vi "Draw Shade.vi"(8 "error in (no error)":errorcluster, 11 "ScrollingList in":refnum<class "ScrollingList.lvclass">) -> (0 "error out":errorcluster, 3 "ScrollingList out":refnum<class "ScrollingList.lvclass">)   [LabVIEW 2020, in "ScrollingList.lvclass"]
uses:
  ScrollingList.lvclass
  C:/Program Files/National Instruments/LabVIEW 2020/vi.lib/QSI/QControls/QControl Classes/Picture/Picture.lvclass
  ScrollingList.lvclass/ScrollingList.ctl
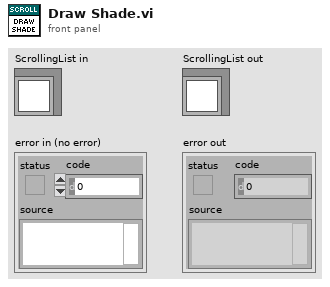
[diagram p1: front panel]
types:
  T1 = cluster{"left":i16, "top":i16, "right":i16, "bottom":i16}
  T2 = cluster{"Width":u16, "Style":enum32{"Solid", "Dash", "Dot", "DashDot", "DashDotDot"}}
  T3 = typedef "ScrollingList.lvclass/State Data.ctl" = cluster{"Timeout":i32, "Time":timestamp, "Y":i32, "Origin:Top":i16, "Rate":dbl, "ListItems":string[], "Item Height":i32, "Max Height":i32}
  T4 = typedef "LVBoundsTypeDef.ctl" = cluster{"Width":u32, "Height":u32}
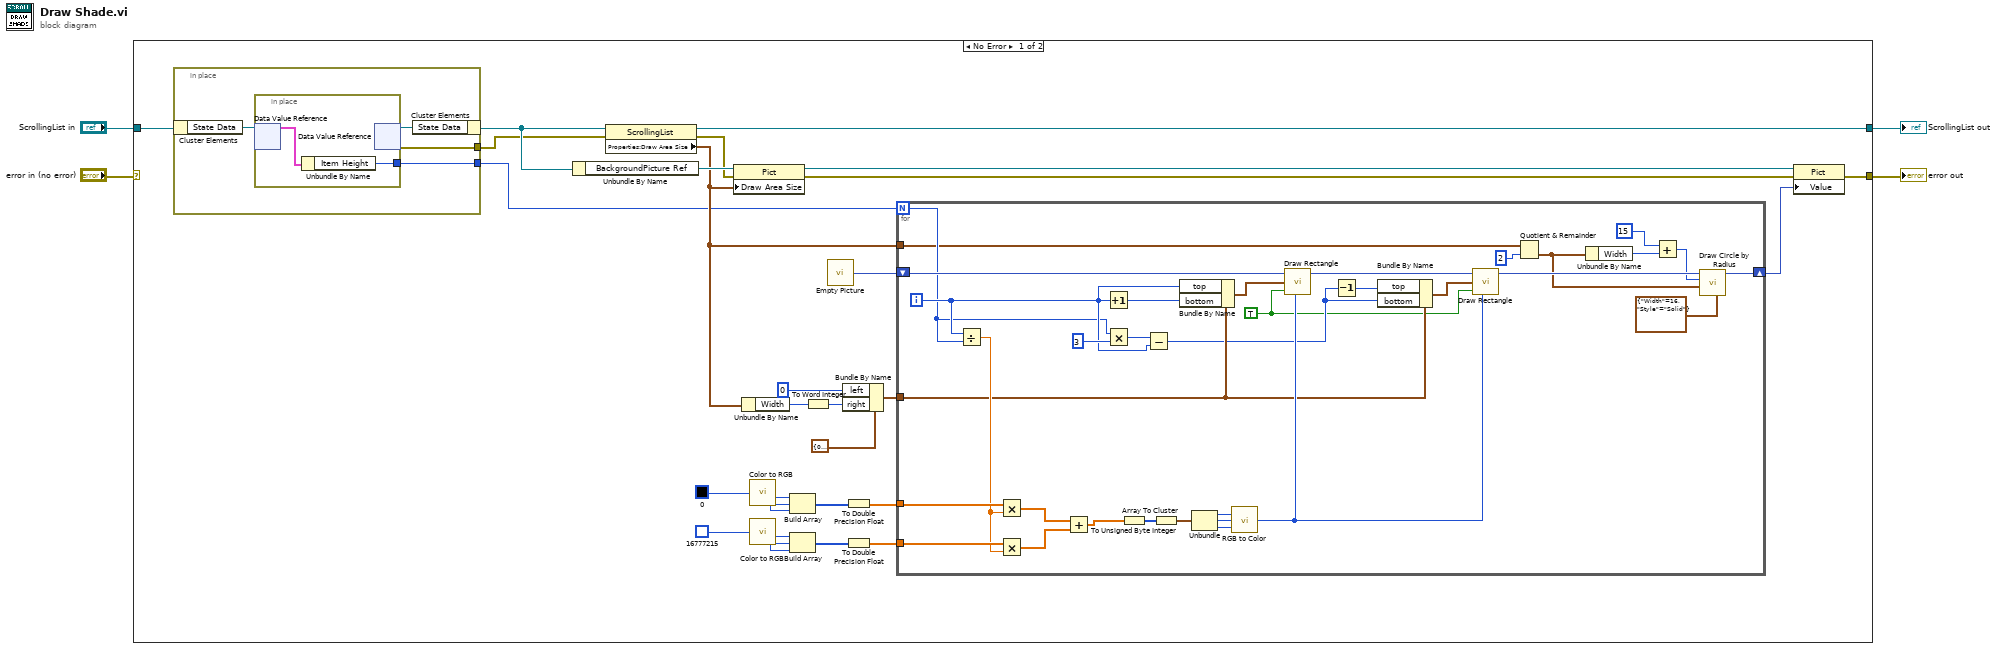
[diagram p0: block diagram]
diagram:
  n1 = case shown="No Error" "error in (no error)" {
    selector: "error in (no error)" -> [_ w76]
    tunnel: [w5 w76] -> w3
    tunnel: [w32 w75] -> w1
    tunnel: "ScrollingList in" -> [w34 w75]
    frame No Error {
      n2 = in-place {
        in-place-border: [w37] -> w10
        in-place-border: [w35] -> w31
        n3 = in-place-cluster #1(w34) -> ("State Data"=w38:refnum<data-value>)
        n4 = in-place {
          in-place-border: [w39] -> w37
          n5 = in-place-dvr #2(w38) -> (w40:T3)  [unwired: 1 out]
          n6 = Unbundle By Name(w40) -> ("Item Height"=w39:i32)
          n7 = in-place-dvr #2() -> (w36:refnum<data-value>, w35:errorcluster)  [unwired: 1 in]
        }
        n8 = in-place-cluster #1("State Data"=w36) -> (w33:refnum<class "ScrollingList.lvclass">)
      }
      n9 = Unbundle By Name(w33) -> ("BackgroundPicture Ref"=w30:refnum<vi>)
      n10 = property class="ScrollingList"(reference=w33, error in=w31) -> (reference out=w32:refnum<class "ScrollingList.lvclass">, error out=w8:errorcluster, "Properties:Draw Area Size"=w11:T4)
      n11 = property class="Pict"(reference=w30, error in=w8, "Draw Area Size"=w11) -> (reference out=w9:refnum<vi>, error out=w7:errorcluster)
      n12 = Unbundle By Name(w11) -> ("Width"=w29:u32)
      n13 = call <vilib>:"Color to RGB.vi"("Color"=u32 0) -> ("R"=w24:u8, "G"=w23:u8, "B"=w22:u8)  [unwired: 1 out]
      n14 = call <vilib>:"Color to RGB.vi"("Color"=u32 16777215) -> ("R"=w20:u8, "G"=w19:u8, "B"=w18:u8)  [unwired: 1 out]
      n15 = Build Array(w24, w23, w22) -> (w21:u8[])
      n16 = Build Array(w20, w19, w18) -> (w17:u8[])
      n17 = To Word Integer(number=w29) -> (16bit integer=w12:i16)
      n18 = call "Empty Picture"() -> ("empty picture"=w25:picture)
      n19 = Bundle By Name(cluster=T1 {"left"=0, "top"=0, "right"=0, "bottom"=0} ("rect"), "left"=i16 0, "right"=w12) -> (w27:T1)
      n20 = To Double Precision Float(number=w21) -> (double precision float=w14:dbl[])
      n21 = To Double Precision Float(number=w17) -> (double precision float=w13:dbl[])
      n22 = for {
        N: w10 -> [w53]
        tunnel: w27 -> [w54]
        shift-right: [w45] -> w6
        shift-left: w25 -> [w74]
        tunnel: w14 -> [w66]
        tunnel: w13 -> [w65]
        tunnel: w11 -> [w48]
        i -> [w56]
        w50 = TRUE ("fill?(F)")
        n23 = Divide(x=w56, y=w53) -> (x/y=w62:dbl)
        n24 = Multiply(x=w66, y=w62) -> (x*y=w64:dbl[])
        n25 = Multiply(x=w65, y=w62) -> (x*y=w63:dbl[])
        n26 = Add(x=w64, y=w63) -> (x+y=w61:dbl[])
        n27 = Increment(x=w56) -> (x+1=w72:i32)
        n28 = Multiply(x=w53, y=3) -> (x*y=w57:i32)
        n29 = To Unsigned Byte Integer(number=w61) -> (unsigned 8bit integer=w67:u8[])
        n30 = Subtract(x=w57, y=w56) -> (x-y=w51:i32)
        n31 = Array To Cluster(array=w67) -> (cluster=w68:cluster{"[0]":u8, "[1]":u8, "[2]":u8})
        n32 = Bundle By Name(cluster=w54, "top"=w56, "bottom"=w72) -> (w73:T1)
        n33 = Unbundle(w68) -> ("[0]"=w69:u8, "[1]"=w70:u8, "[2]"=w71:u8)
        n34 = call <vilib>:"RGB to Color.vi"("B"=w71, "G"=w70, "R"=w69) -> ("Color"=w59:u32)
        n35 = call <vilib>:"Draw Rectangle.vi"("picture"=w74, "rect"=w73, "fill?(F)"=w50, "color(black)"=w59) -> ("new picture"=w60:picture)  [unwired: 5 in]
        n36 = Decrement(x=w51) -> (x-1=w52:i32)
        n37 = Bundle By Name(cluster=w54, "top"=w52, "bottom"=w51) -> (w55:T1)
        n38 = call <vilib>:"Draw Rectangle.vi"("picture"=w60, "rect"=w55, "fill?(F)"=w50, "color(black)"=w59) -> ("new picture"=w49:picture)  [unwired: 5 in]
        n39 = Quotient & Remainder(x=w48, y=u32 2) -> (floor(x/y)=w46:T4)  [unwired: 1 out]
        n40 = Unbundle By Name(w46) -> ("Width"=w43:u32)
        n41 = Add(x=u32 15, y=w43) -> (x+y=w42:u32)
        n42 = call <vilib>:"Draw Circle by Radius.vi"("pen"=T2 {"Width"=16, "Style"=enum."Solid"}, "pixel center"=w46, "radius"=w42, "picture"=w49) -> ("new picture"=w45:picture)  [unwired: 7 in]
      }
      n43 = property class="Pict"(reference=w9, error in=w7, "Value"=w6) -> (error out=w5:errorcluster)  [unwired: 1 out]
    }
    frame Error {
    }
  }
  "error out" <- w3
  "ScrollingList out" <- w1
